vi "Configure Trigger Source.vi"(7 "Trigger External (T)":bool=TRUE, 8 "error in (no error)":errorcluster, 11 "VISA resource name":refnum<visa-resource-name>) -> (0 "error out":errorcluster, 3 "VISA resource name out":refnum<visa-resource-name>)   [LabVIEW 2020, in "QuPMXdriver.lvlib"]
doc: "Configures trigger source to external or internal."
uses:
  QuPMXdriver.lvlib
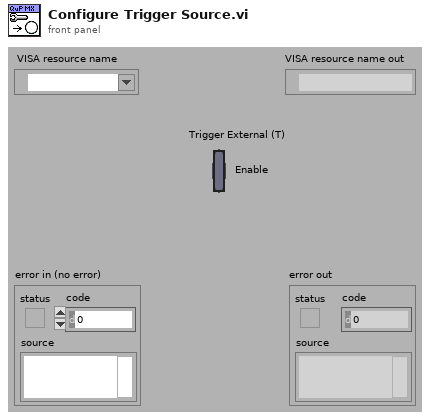
[diagram p1: front panel]
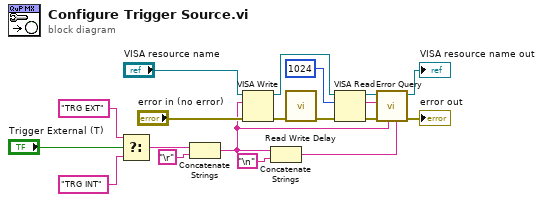
[diagram p0: block diagram]
diagram:
  n1 = Select(t="TRG EXT" ("write buffer"), s="Trigger External (T)", f="TRG INT" ("write buffer")) -> (s? t:f=w12:string)
  n2 = Concatenate Strings(w12, "\r") -> (w2:string)
  n3 = VISA Write(VISA resource name="VISA resource name", write buffer=w2, error in (no error)="error in (no error)") -> (VISA resource name out=w7:refnum<visa-resource-name>, error out=w6:errorcluster)  [unwired: 1 out]
  n4 = Concatenate Strings(w2, "\n") -> (w1:string)
  n5 = call "Read Write Delay.vi"("error in"=w6) -> ("error out"=w10:errorcluster)  [unwired: 10 in]
  n6 = VISA Read(VISA resource name=w7, byte count=u32 1024, error in (no error)=w10) -> (VISA resource name out=w8:refnum<visa-resource-name>, read buffer=w4:string, error out=w5:errorcluster)  [unwired: 1 out]
  n7 = call "Error Query.vi"("Expected read buffer"=w1, "Last command"=w2, "error in (no error)"=w5, "Read buffer"=w4, "VISA resource name"=w8) -> ("error out"=→"error out":errorcluster, "VISA resource name out"=→"VISA resource name out":refnum<visa-resource-name>)  [unwired: 5 in]
